vi "Stop Client.vi"(8 "error in":errorcluster, 11 "NATS Client":refnum<class "NATS Client.lvclass">) -> (0 "error out":errorcluster)   [LabVIEW 2024, in "NATS Client.lvlib" / "NATS Client.lvclass"]
doc: "Stops the Client asynchronous daemon."
uses:
  NATS Client.lvclass
  NATS Client.lvclass/NATS Client.ctl
  get async stop notifier.vi
  Get Connection DVR.vi
  get subscriptions queue.vi
  Get subscription map.vi
  Get error queue.vi
  NATS Subscription/NATS Subscription.lvclass
  <vilib>/NATS/NATS Core/NATS Core.lvlib
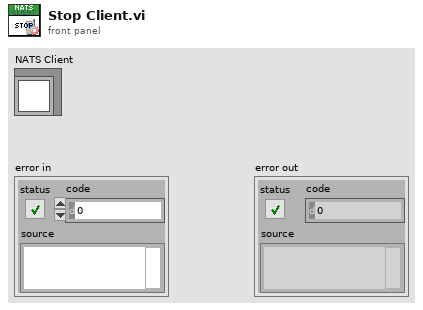
[diagram p1: front panel]
types:
  T1 = typedef "NATS Core.lvlib/nats connection.ctl" = cluster{"connection ID":refnum<k5>, "server INFO":string, "timeout ms":i32, "verbose?":bool, "server headers?":bool, "client headers?":bool}
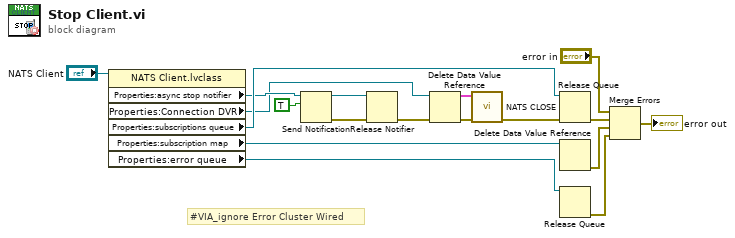
[diagram p0: block diagram]
diagram:
  # "#VIA_ignore Error Cluster Wired"
  n1 = property on="Property Node" class="NATS Client.lvclass"(reference="NATS Client") -> ("Properties:async stop notifier"=w16:refnum<notifier>, "Properties:Connection DVR"=w13:refnum<data-value>, "Properties:subscriptions queue"=w17:refnum<queue>, "Properties:subscription map"=w10:refnum<data-value>, "Properties:error queue"=w11:refnum<queue>)  [unwired: 1 in, 2 out]
  n2 = Send Notification(notification=TRUE, notifier=w16) -> (notifier out=w2:refnum<notifier>, error out=w9:errorcluster)  [unwired: 1 in]
  n3 = Release Notifier(notifier=w2, error in (no error)=w9) -> (error out=w3:errorcluster)  [unwired: 1 in, 2 out]
  n4 = Delete Data Value Reference(data value reference=w13, error in=w3) -> (data value=w14:T1, error out=w15:errorcluster)
  n5 = call <vilib>:"NATS CLOSE.vi"("error in"=w15, "nats connection in"=w14) -> ("error out"=w1:errorcluster)  [unwired: 9 in]
  n6 = Release Queue(queue=w17, error in (no error)=w1) -> (error out=w8:errorcluster)  [unwired: 1 in, 2 out]
  n7 = Delete Data Value Reference(data value reference=w10) -> (error out=w7:errorcluster)  [unwired: 1 in, 1 out]
  n8 = Release Queue(queue=w11) -> (error out=w6:errorcluster)  [unwired: 2 in, 2 out]
  n9 = Merge Errors("error in", w8, w7, w6) -> (→"error out":errorcluster)
